vi "ConvertAction.vi"(1 "RAW cluster 2":cluster{i16[][]}[](array[cluster])=[{[[0, 0, 0, 0, 0, 0, 0, 0], [0, 0, 0, 0, 0, 0, 0, 0]]}, {[[0, 0, 0, 0, 0, 0, 0, 0], [0, 0, 0, 0, 0, 0, 0, 0]]}, {[[0, 0, 0, 0, 0, 0, 0, 0], [0, 0, 0, 0, 0, 0, 0, 0]]}], 2 "Macro Info 2D 2":T4(array[cluster])=[{"Duration (s)"=0.01, "Instruction Description"="MCP select", "Input Bits"=[], "Output Bits"=[FALSE, FALSE, FALSE, TRUE, FALSE, FALSE, FALSE, FALSE, FALSE, FALSE, FALSE, FALSE, FALSE, FALSE, FALSE, FALSE, FALSE, FALSE, FALSE, FALSE, FALSE, FALSE, FALSE, FALSE, FALSE, FALSE, FALSE, FALSE, FALSE, FALSE, FALSE, FALSE, FALSE, FALSE, FALSE, FALSE, FALSE, FALSE], "Excitations"=[0.00012004561733458713, -0.00044621153090514343, -0.0003202049311559398, 0.0, -0.0003733656916932801, -0.00011331671354867952, -0.0004071009076348105, -0.00010699120666020263, -0.00016683684024371525, -0.00024630049992344717, -0.00034726627977641394, 0.0, 0.0, 0.0, 0.0, 0.0], "Steps"=1, "Changes"=[TRUE, FALSE]}, {"Duration (s)"=0.1, "Instruction Description"="MCP out", "Input Bits"=[], "Output Bits"=[FALSE, FALSE, FALSE, FALSE, FALSE, TRUE, FALSE, FALSE, FALSE, FALSE, FALSE, FALSE, FALSE, FALSE, FALSE, FALSE, FALSE, FALSE, FALSE, FALSE, FALSE, FALSE, FALSE, FALSE, FALSE, FALSE, FALSE, FALSE, FALSE, FALSE, FALSE, FALSE, FALSE, FALSE, FALSE, FALSE, FALSE, FALSE], "Excitations"=[0.00012004561733458713, -0.00044621153090514343, -0.0003202049311559398, 0.0, -0.0003733656916932801, -0.00011331671354867952, -0.0004071009076348105, -0.00010699120666020263, -0.00016683684024371525, -0.00024630049992344717, -0.00034726627977641394, 0.0, 0.0, 0.0, 0.0, 0.0], "Steps"=1, "Changes"=[TRUE, FALSE]}, {"Duration (s)"=1.0, "Instruction Description"="wait 3 s", "Input Bits"=[], "Output Bits"=[FALSE, FALSE, FALSE, FALSE, FALSE, FALSE, FALSE, FALSE, FALSE, FALSE, FALSE, FALSE, FALSE, FALSE, FALSE, FALSE, FALSE, FALSE, FALSE, FALSE, FALSE, FALSE, FALSE, FALSE, FALSE, FALSE, FALSE, FALSE, FALSE, FALSE, FALSE, FALSE, FALSE, FALSE, FALSE, FALSE, FALSE, FALSE], "Excitations"=[0.00012004561733458713, -0.00044621153090514343, -0.0003202049311559398, 0.0, -0.0003733656916932801, -0.00011331671354867952, -0.0004071009076348105, -0.00010699120666020263, -0.00016683684024371525, -0.00024630049992344717, -0.00034726627977641394, 0.0, 0.0, 0.0, 0.0, 0.0], "Steps"=1, "Changes"=[TRUE, FALSE]}], 3 "Instructions per Action":i32=3) -> (0 "RT Action":T1={"Macro Instructions"=[{"Duration (s)"=0.01, "Steps"=1, "Changes"=[TRUE, FALSE], "Triggers"=[FALSE, FALSE, FALSE, TRUE, FALSE, FALSE, FALSE, FALSE, FALSE, FALSE, FALSE, FALSE, FALSE, FALSE, FALSE, FALSE, FALSE, FALSE, FALSE, FALSE, FALSE, FALSE, FALSE, FALSE, FALSE, FALSE, FALSE, FALSE, FALSE, FALSE, FALSE, FALSE, FALSE, FALSE, FALSE, FALSE, FALSE, FALSE], "RAW cmds 2D"=[[0, 0, 0, 0, 0, 0, 0, 0], [0, 0, 0, 0, 0, 0, 0, 0]]}, {"Duration (s)"=0.1, "Steps"=1, "Changes"=[TRUE, FALSE], "Triggers"=[FALSE, FALSE, FALSE, FALSE, FALSE, TRUE, FALSE, FALSE, FALSE, FALSE, FALSE, FALSE, FALSE, FALSE, FALSE, FALSE, FALSE, FALSE, FALSE, FALSE, FALSE, FALSE, FALSE, FALSE, FALSE, FALSE, FALSE, FALSE, FALSE, FALSE, FALSE, FALSE, FALSE, FALSE, FALSE, FALSE, FALSE, FALSE], "RAW cmds 2D"=[[0, 0, 0, 0, 0, 0, 0, 0], [0, 0, 0, 0, 0, 0, 0, 0]]}, {"Duration (s)"=1.0, "Steps"=1, "Changes"=[TRUE, FALSE], "Triggers"=[FALSE, FALSE, FALSE, FALSE, FALSE, FALSE, FALSE, FALSE, FALSE, FALSE, FALSE, FALSE, FALSE, FALSE, FALSE, FALSE, FALSE, FALSE, FALSE, FALSE, FALSE, FALSE, FALSE, FALSE, FALSE, FALSE, FALSE, FALSE, FALSE, FALSE, FALSE, FALSE, FALSE, FALSE, FALSE, FALSE, FALSE, FALSE], "RAW cmds 2D"=[[0, 0, 0, 0, 0, 0, 0, 0], [0, 0, 0, 0, 0, 0, 0, 0]]}], "Slow AO Array"=[], "Duration (s)"=1.11, "Toggle"=FALSE} {"Slow AO Array"."Duration, Gain, NewVal" format="%#_3g"})   [LabVIEW 2018]
uses:
  ActionCluster.ctl
  Instructions_RT.ctl
  ParameterSubCluster.ctl
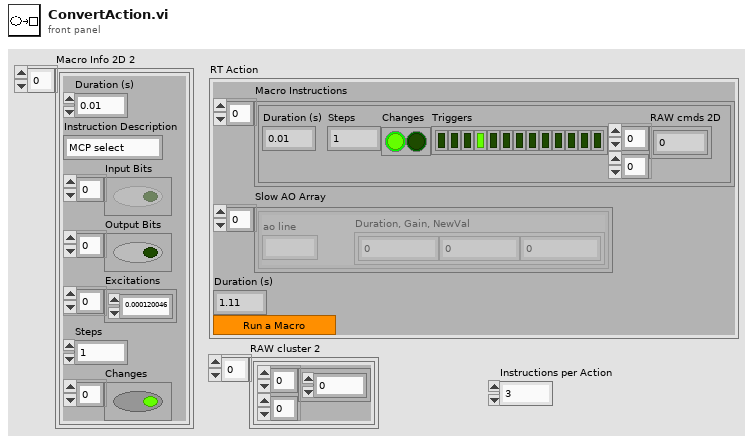
[diagram p1: front panel]
types:
  T1 = typedef "ActionCluster.ctl" = cluster{"Macro Instructions":T2, "Slow AO Array":T3, "Duration (s)":dbl, "Toggle":bool}
  T2 = typedef "Instructions_RT.ctl" = cluster{"Duration (s)":dbl, "Steps":i32, "Changes":bool[], "Triggers":bool[], "RAW cmds 2D":i16[][]}[]
  T3 = typedef "ParameterSubCluster.ctl" = cluster{"ao line":string, "Duration, Gain, NewVal":dbl[]}[]
  T4 = cluster{"Duration (s)":dbl, "Instruction Description":string, "Input Bits":bool[], "Output Bits":bool[], "Excitations":dbl[], "Steps":i32, "Changes":bool[]}[]
  T5 = cluster{"Duration (s)":dbl, "Steps":i32, "Changes":bool[], "Triggers":bool[], "RAW cmds 2D":i16[][]}
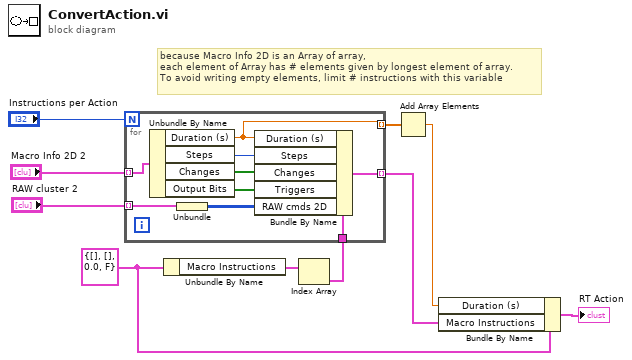
[diagram p0: block diagram]
diagram:
  w4 = T1 {"Macro Instructions"=[], "Slow AO Array"=[], "Duration (s)"=0.0, "Toggle"=FALSE} ("RT Action")
  # "because Macro Info 2D is an Array of array, \neach element of Array has # elements given by longest element of array.\nTo avoid writing empty elements, limit # instructions with this variable"
  n1 = Unbundle By Name(w4) -> ("Macro Instructions"=w10:T2)
  n2 = Index Array(array=w10) -> (element=w9:T5)  [unwired: 1 in]
  n3 = for {
    N: "Instructions per Action" -> [_]
    tunnel: w9 -> [w19]
    tunnel: [w18] -> w8 mode=indexing
    tunnel: "RAW cluster 2" -> [w17] mode=indexing
    tunnel: "Macro Info 2D 2" -> [w15] mode=indexing
    tunnel: [w11] -> w2 mode=indexing
    n4 = Unbundle By Name(w15) -> ("Duration (s)"=w11:dbl, "Steps"=w14:i32, "Changes"=w13:bool[], "Output Bits"=w12:bool[])
    n5 = Unbundle(w17) -> (w16:i16[][])
    n6 = Bundle By Name(cluster=w19, "Duration (s)"=w11, "Steps"=w14, "Changes"=w13, "Triggers"=w12, "RAW cmds 2D"=w16) -> (w18:T5)
  }
  n7 = Add Array Elements(numeric array=w2) -> (sum=w1:dbl)
  n8 = Bundle By Name(cluster=w4, "Duration (s)"=w1, "Macro Instructions"=w8) -> (→"RT Action":T1)
